vi "NIVS.Channels.Read.vi"(8 "error in (no error)":errorcluster, 11 "State Variables":T1) -> (0 "error out":errorcluster)   [LabVIEW 2015]
uses:
  Types/Main.StateVariables.ctl
  <vilib>/Utility/miscctls.llb/LVPositionTypeDef.ctl
  Types/Execute.UserEventRefs.ctl
  <vilib>/NI Veristand/Execution/Workspace/SystemStateRegEventRef.ctl
  <vilib>/NI Veristand/Execution/Workspace/Target State Info.ctl
  <vilib>/NI Veristand/Execution/Workspace/Target State.ctl
  <vilib>/NI Veristand/Execution/WaveformStreaming/Waveform Data Watcher Event Data (DBL).ctl
  <vilib>/NI Veristand/Execution/WaveformStreaming/WaveformStreamSpecification.ctl
  NationalInstruments.VeriStand.ClientAPI
  <vilib>/NI Veristand/Execution/Workspace/SystemStateEventRef.ctl
  <vilib>/NI Veristand/Execution/Workspace/WorkspaceAPI.ctl
  Types/UI.Object.ctl
  Types/Waveforms.Info.ctl
  <vilib>/NI Veristand/Execution/WaveformStreaming/Registered Waveform Streams Data Event Refnum (DBL).ctl
  <vilib>/NI Veristand/Execution/WaveformStreaming/WaveformDataWatcherDBL.ctl
  <vilib>/NI Veristand/Execution/WaveformStreaming/WaveformStreamingAPI.ctl
  <vilib>/NI Veristand/Execution/Workspace/NI VeriStand - Get Multiple Channel Values.vi
  <vilib>/NI Veristand/Execution/Workspace/NI_VS Workspace ExecutionAPI.lvlib
  <vilib>/NI Veristand/Execution/WaveformStreaming/NI_VS Waveform Streaming Interface.lvlib
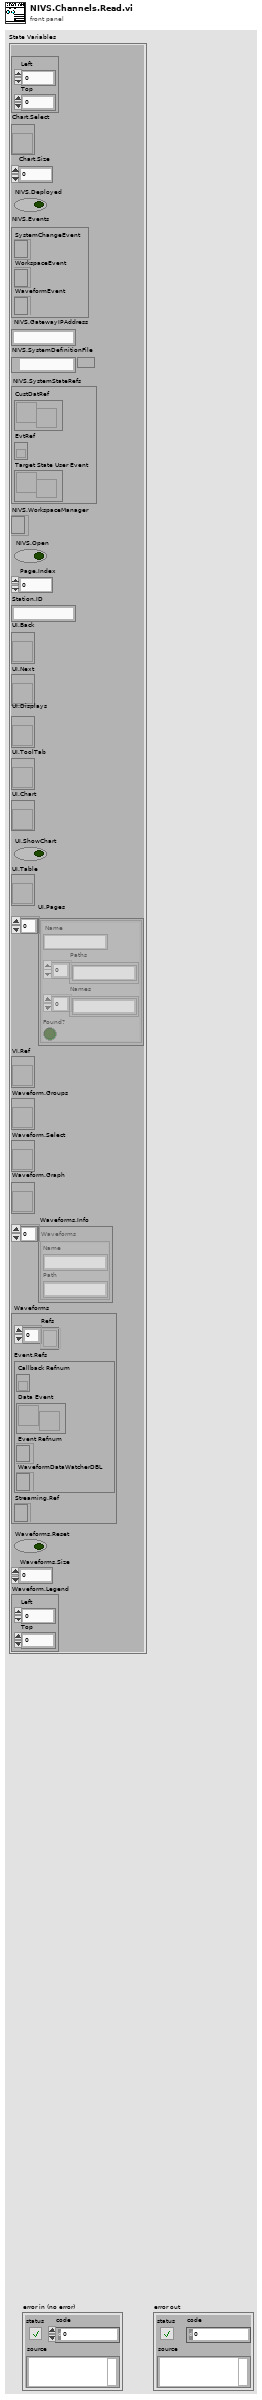
[diagram p1: front panel]
types:
  T1 = typedef "Main.StateVariables.ctl" = cluster{"Chart.Legend":T2, "Chart.Select":refnum<vi>, "Chart.Size":i32, "NIVS.Deployed":bool, "NIVS.Events":T3, "NIVS.GatewayIPAddress":string, "NIVS.SystemDefinitionFile":path, "NIVS.SystemStateRefs":T5, "NIVS.WorkspaceManager":T6, "NIVS.Open":bool, "Page.Index":u32, "Station.ID":string, "UI.Back":refnum<vi>, "UI.Next":refnum<vi>, "UI.Displays":refnum<vi>, "UI.ToolTab":refnum<vi>, "UI.Chart":refnum<vi>, "UI.ShowChart":bool, "UI.Table":refnum<vi>, "UI.Pages":T7[], "VI.Ref":refnum<vi>, "Waveform.Groups":refnum<vi>, "Waveform.Select":refnum<vi>, "Waveform.Graph":refnum<vi>, "Waveforms.Info":T8[], "Waveforms":cluster{"Refs":T9[], "Event.Refs":T10, "Streaming.Ref":T12}, "Waveforms.Reset":bool, "Waveforms.Size":i32, "Waveform.Legend":T2}
  T2 = typedef "LVPositionTypeDef.ctl" = cluster{"Left":i32, "Top":i32}
  T3 = typedef "Execute.UserEventRefs.ctl" = cluster{"SystemChangeEvent":T4, "WorkspaceEvent":refnum<event-registration>, "WaveformEvent":refnum<event-registration>}
  T4 = typedef "NI_VS Workspace ExecutionAPI.lvlib/SystemStateRegEventRef.ctl" = refnum<event-registration>
  T5 = typedef "NI_VS Workspace ExecutionAPI.lvlib/SystemStateEventRef.ctl" = cluster{"CustDatRef":refnum<user-event>, "EvtRef":refnum<k27>, "Target State User Event":refnum<user-event>}
  T6 = typedef "NI_VS Workspace ExecutionAPI.lvlib/WorkspaceAPI.ctl" = refnum<k24>
  T7 = typedef "UI.Object.ctl" = cluster{"Name":string, "Paths":string[], "Names":string[], "Found?":bool}
  T8 = typedef "Waveforms.Info.ctl" = cluster{"Name":string, "Path":string}
  T9 = typedef "NI_VS Waveform Streaming Interface.lvlib/WaveformStreamSpecification.ctl" = refnum<k24>
  T10 = typedef "NI_VS Waveform Streaming Interface.lvlib/Registered Waveform Streams Data Event Refnum (DBL).ctl" = cluster{"Callback Refnum":refnum<k27>, "Data Event":refnum<user-event>, "Event Refnum":refnum<event-registration>, "WaveformDataWatcherDBL":T11}
  T11 = typedef "NI_VS Waveform Streaming Interface.lvlib/WaveformDataWatcherDBL.ctl" = refnum<k24>
  T12 = typedef "NI_VS Waveform Streaming Interface.lvlib/WaveformStreamingAPI.ctl" = refnum<k24>
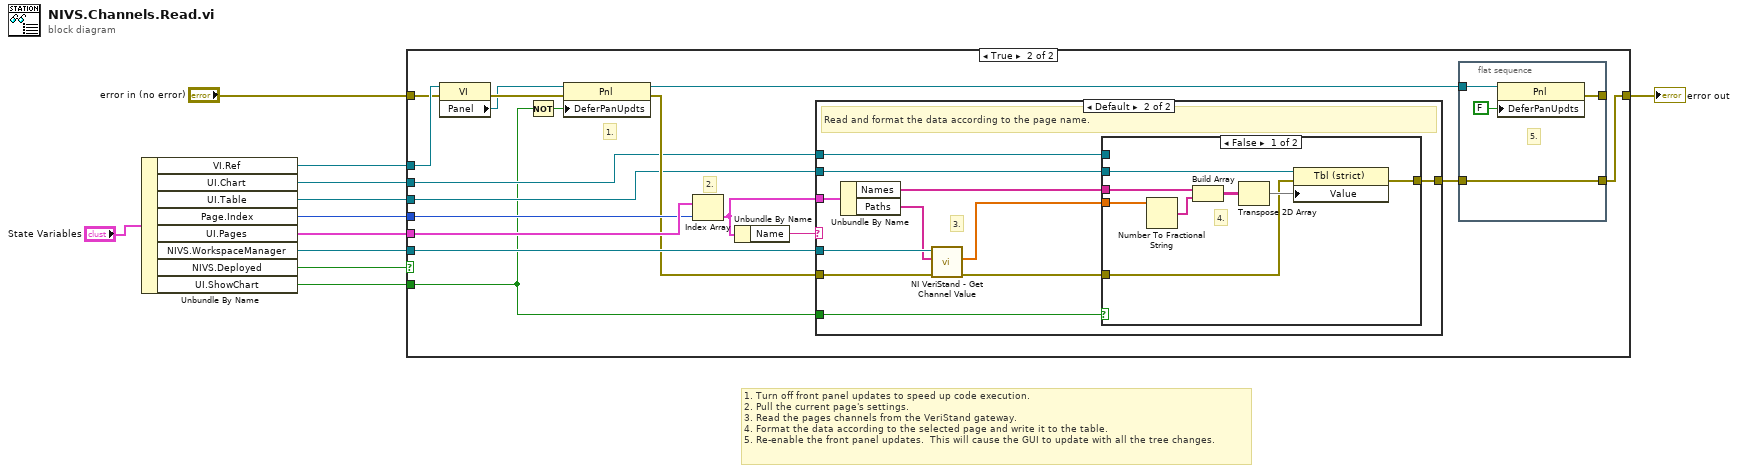
[diagram p0: block diagram]
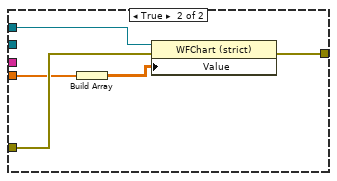
[diagram p4: hidden frame]
diagram:
  # "1. Turn off front panel updates to speed up code execution.\n2. Pull the current page's settings.\n3. Read the pages channels from the VeriStand gateway.\n4. Format the data according to the selected page and write it to the table.\n5. Re-enable the front panel updates.  This will cause the GUI to update with all the tree changes."
  n1 = Unbundle By Name("State Variables") -> ("VI.Ref"=w6:refnum<vi>, "UI.Chart"=w2:refnum<vi>, "UI.Table"=w3:refnum<vi>, "Page.Index"=w5:u32, "UI.Pages"=w4:T7[], "NIVS.WorkspaceManager"=w11:T6, "NIVS.Deployed"=w10:bool, "UI.ShowChart"=w1:bool)
  n2 = case shown="True" w10 {
    tunnel: "error in (no error)" -> [w12 w24]
    tunnel: w4 -> [_ w29]
    tunnel: [w12 w22] -> w9
    tunnel: w11 -> [_ w28]
    tunnel: w6 -> [_ w25]
    tunnel: w5 -> [_ w18]
    tunnel: w3 -> [_ w16]
    tunnel: w2 -> [_ w15]
    tunnel: w1 -> [_ w13]
    frame False {
    }
    frame True {
      # "2."
      # "1."
      n3 = property class="VI"(reference=w25, error in=w24) -> (error out=w27:errorcluster, "Panel"=w26:refnum<vi>)  [unwired: 1 out]
      n4 = Not(x=w13) -> (.not. x?=w14:bool)
      n5 = property class="Pnl"(reference=w26, error in=w27, "DeferPanUpdts"=w14) -> (reference out=w21:refnum<vi>, error out=w17:errorcluster)
      n6 = Index Array(array=w29, index=w18) -> (element=w20:T7)
      n7 = Unbundle By Name(w20) -> ("Name"=w19:string)
      n8 = case shown="Default" w19 {
        tunnel: w20 -> [_ w39]
        tunnel: w17 -> [w34 w38]
        tunnel: w28 -> [_ w45]
        tunnel: [w34 w43] -> w23
        tunnel: w16 -> [_ w37]
        tunnel: w15 -> [_ w35]
        tunnel: w13 -> [_ w36]
        frame "OSCOPE" {
          # "OSCOPE page selected.  VS waveforms are handled differently.  Do nothing."
        }
        frame Default {
          # "3."
          # "Read and format the data according to the page name."
          n9 = Unbundle By Name(w39) -> ("Names"=w44:string[], "Paths"=w42:string[])
          n10 = call-poly <vilib>:"NI VeriStand - Get Channel Value.vi"("error in (no error)"=w38, "Channels"=w42, "WorkspaceManager in"=w45) -> ("error out"=w40:errorcluster, "Values"=w41:dbl[])  [unwired: 6 in, 1 out]
          n11 = case shown="False" w36 {
            tunnel: w44 -> [w53 _]
            tunnel: [w52 w55] -> w43
            tunnel: w41 -> [w51 w56]
            tunnel: w40 -> [w47 w58]
            tunnel: w37 -> [w46 _]
            tunnel: w35 -> [_ w57]
            frame False {
              # "4."
              n12 = Number To Fractional String(number=w51) -> (F-format string=w50:string[])  [unwired: 3 in]
              n13 = Build Array(w53, w50) -> (w49:string[][])
              n14 = Transpose 2D Array(2D array=w49) -> (transposed array=w48:string[][])
              n15 = property class="Tbl (strict)"(reference=w46, error in=w47, "Value"=w48) -> (error out=w52:errorcluster)  [unwired: 1 out]
            }
            frame True {
              n16 = Build Array(w56) -> (w54:dbl[][])
              n17 = property class="WFChart (strict)"(reference=w57, error in=w58, "Value"=w54) -> (error out=w55:errorcluster)  [unwired: 1 out]
            }
          }
        }
      }
      n18 = flat-sequence {
        tunnel: w21 -> [w33]
        tunnel: [w32] -> w22
        tunnel: w23 -> [w32]
        tunnel: [w31] -> _
        frame #0 {
          # "5."
          n19 = property class="Pnl"(reference=w33, "DeferPanUpdts"=FALSE ("Defer Panel Updates")) -> (error out=w31:errorcluster)  [unwired: 1 in, 1 out]
        }
      }
    }
  }
  "error out" <- w9
